vi "DWF MSO Query Analog Channel.vi"(0 "Instrument Handle In":u32, 7 "Channel":string, 11 "Error In":errorcluster caption="Error In (no error)") -> (4 "Instrument Handle Out":u32, 6 "Channel Enabled":bool, 8 "Vertical Coupling":i32(ring) items=["AC", "DC"], 10 "Probe Attenuation":i32(ring)=1 items=["1x"=1, "10x"=10], 13 "Vertical Offset":dbl, 14 "Vertical Range":dbl, 15 "Error Out":errorcluster)   [LabVIEW 2015, in "DigilentWF.lvlib"]
doc: "Indicates the vertical configuration of the specified channel."
uses:
  <vilib>/DigilentWF/DigilentWF.lvlib
  dwf.dll
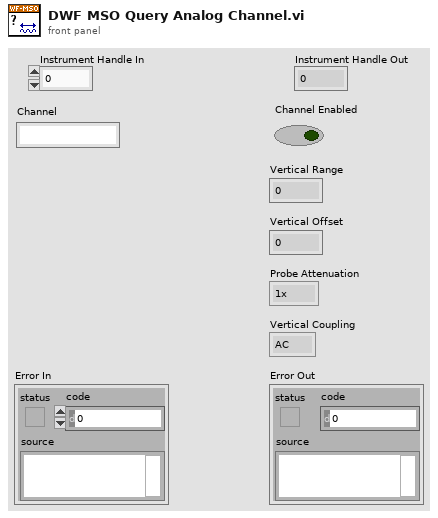
[diagram p1: front panel]
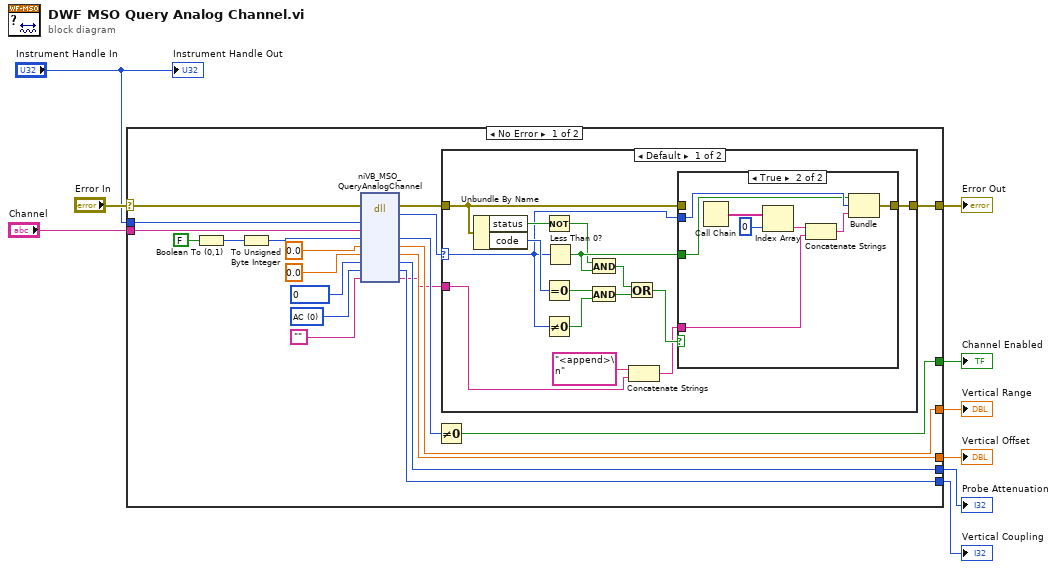
[diagram p0: block diagram]
diagram:
  n1 = case "outter_case" shown="No Error" "Error In" {
    selector: "Error In" -> [w30 w56]
    tunnel: [w27 w56] -> w8
    tunnel: "Instrument Handle In" -> [w26 _]
    tunnel: [w18 _] -> w6
    tunnel: [w16 _] -> w5
    tunnel: [w15 _] -> w4
    tunnel: [w14 _] -> w3
    tunnel: [w13 _] -> w2
    tunnel: "Channel" -> [w10 _]
    frame No Error {
      w19 = 0 items=["AC", "DC"] ("Vertical Coupling")
      w20 = 0 items=["1x"=1, "10x"=10] ("Probe Attenuation")
      n2 = Boolean To (0,1)(Boolean=FALSE ("Channel Enabled")) -> (0, 1=w25:i16)
      n3 = To Unsigned Byte Integer(number=w25) -> (unsigned 8bit integer=w23:u8)
      n4 = dll-call lib="dwf.*" fn="niVB_MSO_QueryAnalogChannel"(error in=w30, "InstrumentHandle"=w26, "Channel"=w10, "ChannelEnabled"=w23, "VerticalRange"=0.0 ("Vertical Range"), "VerticalOffset"=0.0 ("Vertical Offset"), "ProbeAttenuation"=w20, "VerticalCoupling"=w19, "szError"="") -> (error out=w29:errorcluster, "return type"=w28:i32, "ChannelEnabled"=w17:u8, "VerticalRange"=w16:dbl, "VerticalOffset"=w15:dbl, "ProbeAttenuation"=w14:i32, "VerticalCoupling"=w13:i32, "szError"=w11:string)  [unwired: 4 in, 1 out]
      n5 = Not Equal To 0?(x=w17) -> (x != 0?=w18:bool)
      n6 = case "inner_case" shown="Default" w28 {
        selector: w28 -> [w35 _]
        tunnel: w29 -> [w36 w55]
        tunnel: [w32 w55] -> w27
        tunnel: w11 -> [w31 _]
        frame Default {
          n7 = Unbundle By Name(w36) -> ("status"=w40:bool, "code"=w44:i32)
          n8 = Not(x=w40) -> (.not. x?=w43:bool)
          n9 = Equal To 0?(x=w44) -> (x = 0?=w39:bool)
          n10 = Not Equal To 0?(x=w35) -> (x != 0?=w42:bool)
          n11 = Less Than 0?(x=w35) -> (x < 0?=w45:bool)
          n12 = And(x=w43, y=w45) -> (x .and. y?=w41:bool)
          n13 = And(x=w39, y=w42) -> (x .and. y?=w38:bool)
          n14 = Or(x=w41, y=w38) -> (x .or. y?=w37:bool)
          n15 = Concatenate Strings("<append>\n" ("string"), w31) -> (w34:string)
          n16 = case shown="True" w37 {
            tunnel: [w46 w53] -> w32
            tunnel: w35 -> [_ w52]
            tunnel: w45 -> [_ w51]
            tunnel: w36 -> [w46 _]
            tunnel: w34 -> [_ w47]
            frame False {
            }
            frame True {
              n17 = Call Chain() -> (call chain=w50:string[])
              n18 = Index Array(array=w50, index=0) -> (element=w49:string)
              n19 = Concatenate Strings(w49, w47) -> (w54:string)
              n20 = Bundle(w51, "return type"=w52, w54) -> (w53:cluster{bool, "return type":i32, string})  [unwired: 1 out]
            }
          }
        }
        frame 0 {
        }
      }
    }
    frame Error {
    }
  }
  "Error Out" <- w8
  "Channel Enabled" <- w6
  "Vertical Range" <- w5
  "Vertical Offset" <- w4
  "Probe Attenuation" <- w3
  "Vertical Coupling" <- w2
  "Instrument Handle Out" <- "Instrument Handle In"
